vi "标样核查.vi"() -> ()   [LabVIEW 2016, in "斯坦道多参数.lvlib"]
panel:
  out "运行状态":u16(ring) items=["空闲", "水样测试", "标样核查"]
  out "seconds since 1Jan1904":timestamp
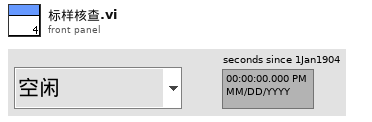
[diagram p1: front panel]
types:
  T1 = cluster{"ph":bool, "DO":bool, "Cond":bool, "Turb":bool, "叶绿素a":bool, "藻密度":bool, "ORP":bool}
  T2 = cluster{"水样数据时间":timestamp, "水样实测值":sgl, "单位":string, "水样数据标识":string, "信号值":sgl, "标样参考值":sgl, "因子编码":string, "探头温度":sgl}
  T3 = cluster{"数据保存间隔":dbl, "保存组数":dbl, "水温标样值":dbl, "pH标样值":dbl, "溶解氧标样值":dbl, "电导率标样值":dbl, "浊度标样值":dbl, "pH启用":bool, "溶解氧启用":bool, "电导率启用":bool, "浊度启用":bool}
  T4 = typedef "LVDateTimeRec.ctl" = cluster{"秒数的小数部分":dbl, "秒":i32, "分":i32, "时":i32, "日":i32, "月":i32, "年":i32, "天数（周）":i32, "天数（年）":i32, "DST":i32}
  T5 = cluster{"温度测量值":sgl, "测量值":sgl, "温度偏移修正值":sgl, "信号值":sgl}
  T6 = cluster{"温度测量值":sgl, "DO%":sgl, "DOmg/L":sgl, "温度偏移修正值":sgl}
  T7 = cluster{"CH":u16, "监测值":dbl, "温度偏移修正值":sgl, "信号值":sgl}
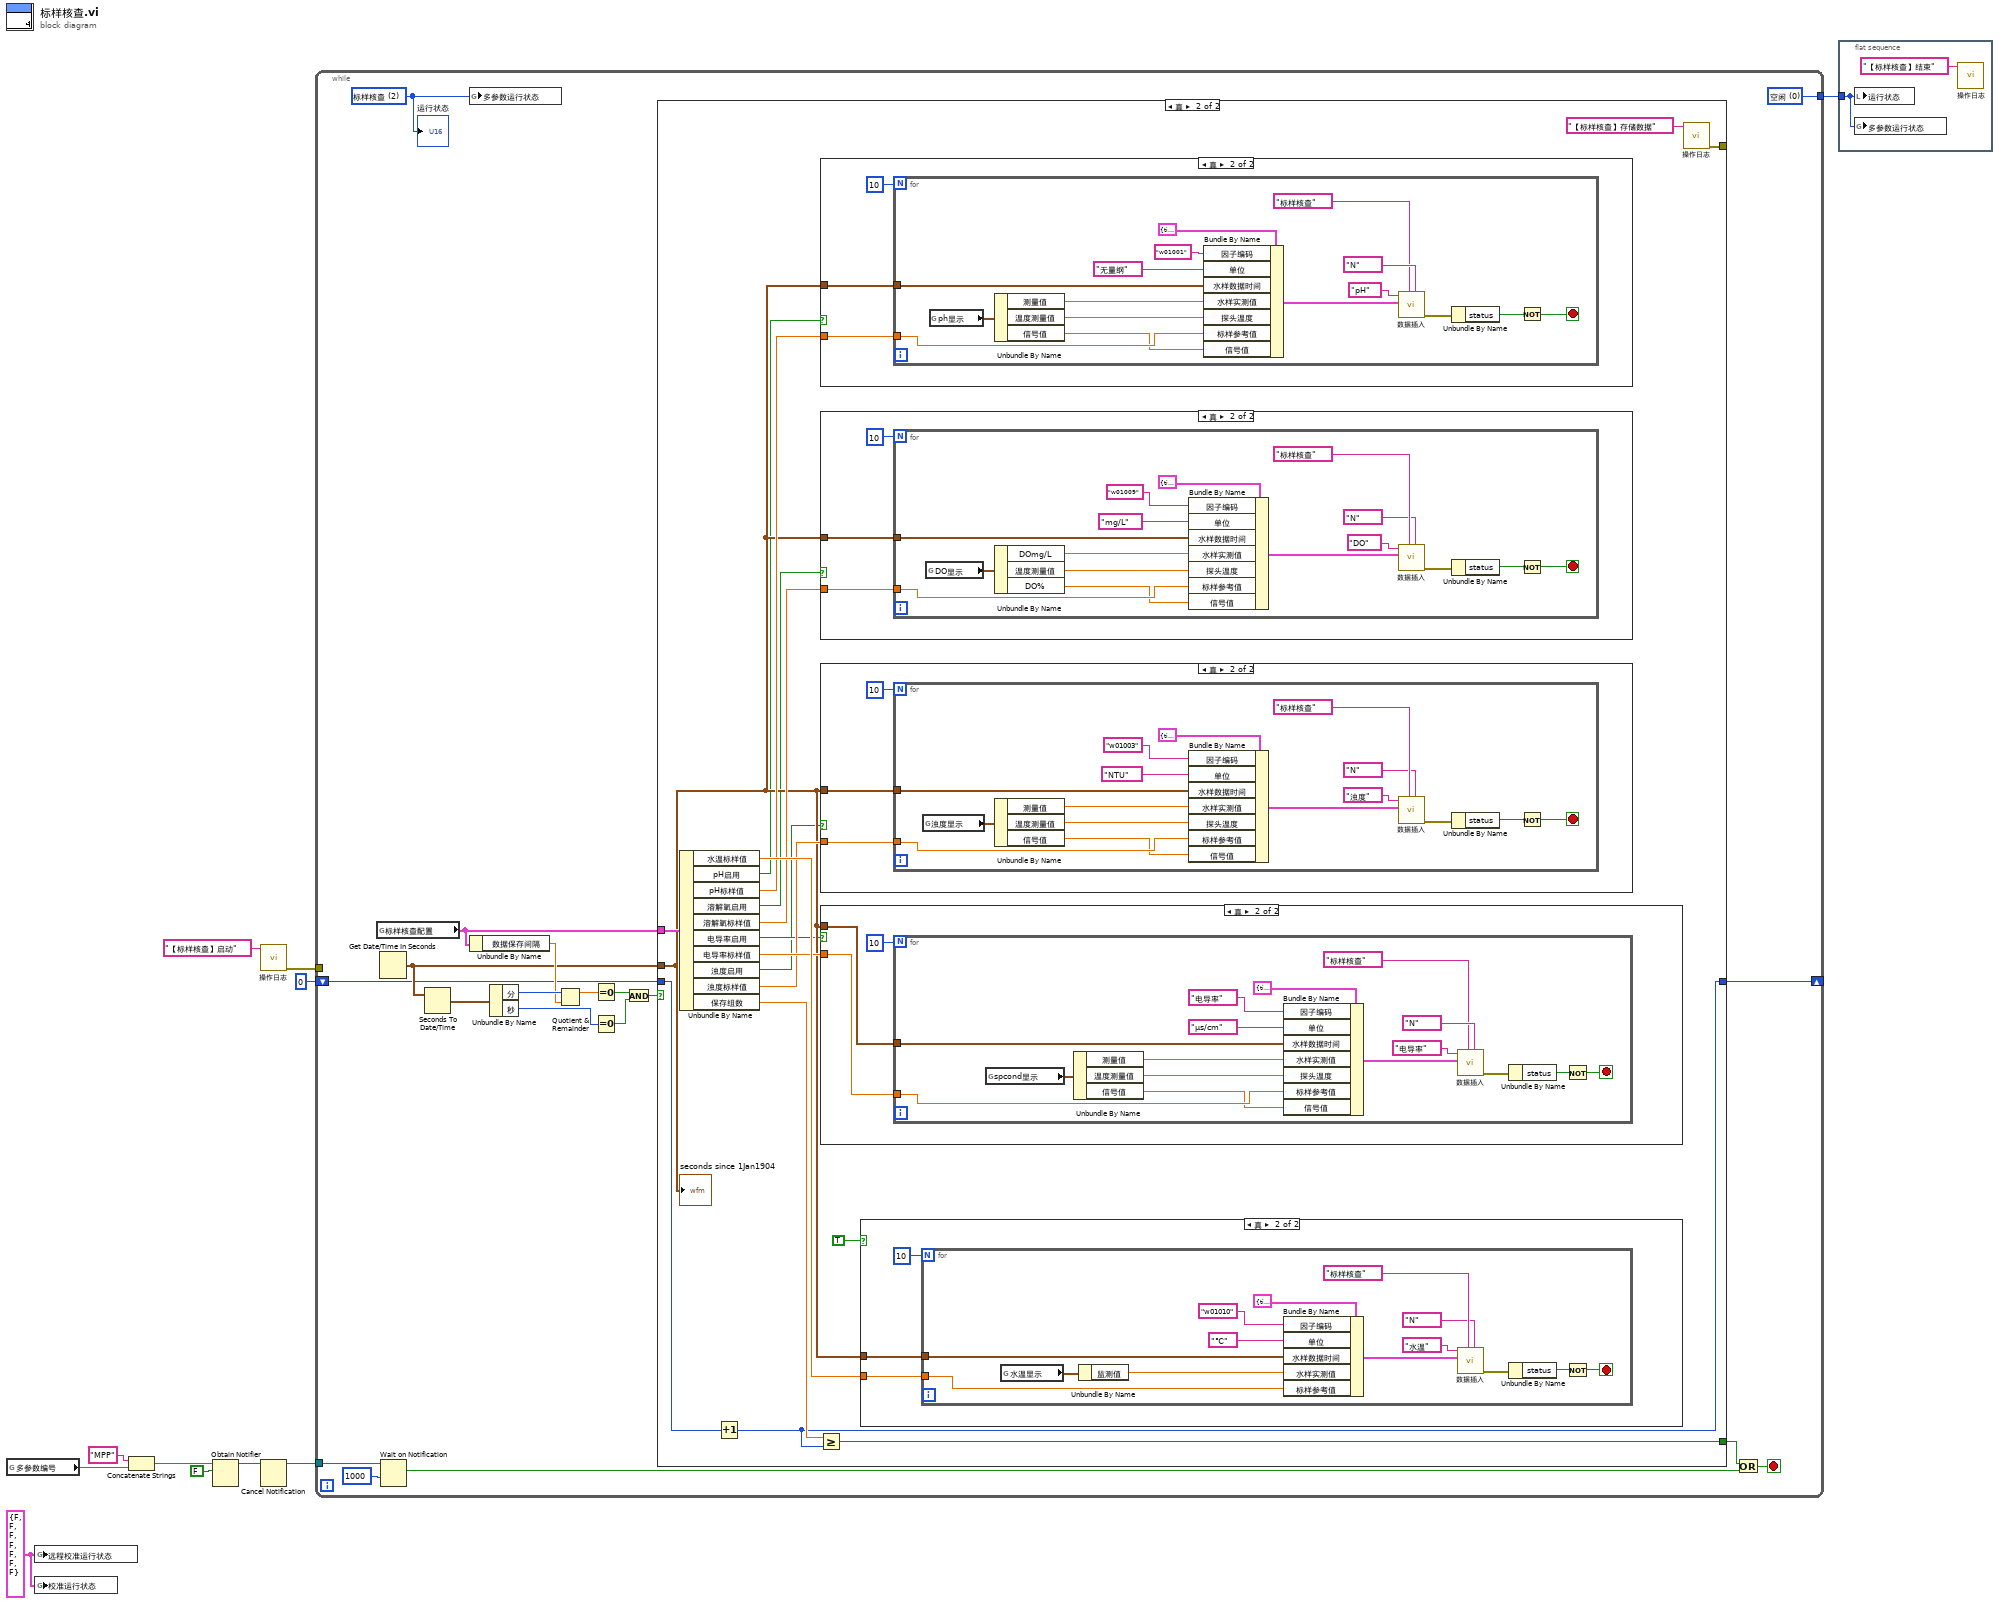
[diagram p0: block diagram]
diagram:
  w2 = T1 {"ph"=FALSE, "DO"=FALSE, "Cond"=FALSE, "Turb"=FALSE, "叶绿素a"=FALSE, "藻密度"=FALSE, "ORP"=FALSE} ("校准运行状态")
  n1 = global read "多参数全局变量.vi" "多参数编号"() -> (w5:string)
  n2 = global write "多参数全局变量.vi" "远程校准运行状态"(w2) -> ()
  n3 = global write "多参数全局变量.vi" "校准运行状态"(w2) -> ()
  n4 = Concatenate Strings("MPP" ("名称（未命名）"), w5) -> (w6:string)
  n5 = Obtain Notifier(name (unnamed)=w6, notification data type=FALSE) -> (notifier out=w9:refnum<notifier>)  [unwired: 2 in, 2 out]
  n6 = call "操作日志.vi"("日志信息"="【标样核查】启动") -> ("error out"=w3:errorcluster)  [unwired: 10 in]
  n7 = Cancel Notification(0:w9) -> (8:w8:refnum<notifier>)  [unwired: 1 in, 2 out]
  n8 = while {
    tunnel: [w21] -> w7
    tunnel: w8 -> [w20]
    tunnel: w3 -> [_]
    shift-right: [w14] -> _
    shift-left: 0 -> [w15]
    stop <- w13 stop-if-true
    w21 = u16 0 items=["空闲", "水样测试", "标样核查"] ("多参数运行状态")
    w17 = u16 2 items=["空闲", "水样测试", "标样核查"] ("多参数运行状态")
    n9 = global read "断电保存变量.vi" "标样核查配置"() -> (w16:T3)
    n10 = Get Date/Time In Seconds() -> (seconds since 1Jan1904=w22:timestamp)
    n11 = Wait on Notification(notifier=w20, timeout in ms (-1)=1000 ("超时毫秒(-1)")) -> (notification=w18:bool)  [unwired: 2 in, 3 out]
    n12 = Seconds To Date/Time(time stamp (now)=w22) -> (date time rec=w30:T4)  [unwired: 1 in]
    n13 = global write "多参数全局变量.vi" "多参数运行状态"(w17) -> ()
    n14 = Unbundle By Name(w16) -> ("数据保存间隔"=w25:dbl)
    n15 = Unbundle By Name(w30) -> ("分"=w26:i32, "秒"=w29:i32)
    n16 = Quotient & Remainder(x=w26, y=w25) -> (x-y*floor(x/y)=w24:dbl)  [unwired: 1 out]
    n17 = Equal To 0?(x=w24) -> (x = 0?=w23:bool)
    n18 = Equal To 0?(x=w29) -> (x = 0?=w28:bool)
    n19 = And(x=w23, y=w28) -> (x .and. y?=w27:bool)
    n20 = case shown="真" w27 {
      tunnel: w16 -> [_ w49]
      tunnel: w22 -> [_ w41]
      tunnel: [_ w42] -> _
      tunnel: w15 -> [w31 w35]
      tunnel: [w31 w33] -> w14
      tunnel: [_ w32] -> w12
      frame False {
      }
      frame True {
        n21 = Unbundle By Name(w49) -> ("水温标样值"=w48:dbl, "pH启用"=w40:bool, "pH标样值"=w47:dbl, "溶解氧启用"=w38:bool, "溶解氧标样值"=w46:dbl, "电导率启用"=w37:bool, "电导率标样值"=w45:dbl, "浊度启用"=w36:bool, "浊度标样值"=w44:dbl, "保存组数"=w34:dbl)
        n22 = Increment(x=w35) -> (x+1=w33:i32)
        n23 = Greater Or Equal?(x=w34, y=w33) -> (x >= y?=w32:bool)
        n24 = case shown="真" w40 {
          tunnel: w47 -> [_ w109]
          tunnel: w41 -> [_ w107]
          frame False {
          }
          frame True {
            n25 = for {
              N: 10 -> [_]
              tunnel: w109 -> [w120]
              tunnel: w107 -> [w113]
              stop <- w114 stop-if-true
              n26 = global read "多参数全局变量.vi" "ph显示"() -> (w119:T5)
              n27 = Unbundle By Name(w119) -> ("测量值"=w118:sgl, "温度测量值"=w117:sgl, "信号值"=w110:sgl)
              n28 = Bundle By Name(cluster=T2 {"水样数据时间"=timestamp(0 s since 1904-01-01), "水样实测值"=0.0, "单位"="", "水样数据标识"="N", "信号值"=0.0, "标样参考值"=0.0, "因子编码"="", "探头温度"=0.0} ("data in"), "因子编码"="w01001", "单位"="无量纲", "水样数据时间"=w113, "水样实测值"=w118, "探头温度"=w117, "标样参考值"=w120, "信号值"=w110) -> (w111:T2)
              n29 = call "数据插入.vi"("数据类型"="N" ("数据标记表"), "测量模式"="标样核查", "data in"=w111, "table输入"="pH") -> ("error out"=w116:errorcluster)  [unwired: 7 in]
              n30 = Unbundle By Name(w116) -> ("status"=w115:bool)
              n31 = Not(x=w115) -> (.not. x?=w114:bool)
            }
          }
        }
        n32 = case shown="真" w38 {
          tunnel: w46 -> [_ w90]
          tunnel: w41 -> [_ w88]
          frame False {
          }
          frame True {
            n33 = for {
              N: 10 -> [_]
              tunnel: w90 -> [w98]
              tunnel: w88 -> [w93]
              stop <- w94 stop-if-true
              n34 = global read "多参数全局变量.vi" "DO显示"() -> (w97:T6)
              n35 = Unbundle By Name(w97) -> ("DOmg/L"=w104:sgl, "温度测量值"=w106:sgl, "DO%"=w91:sgl)
              n36 = Bundle By Name(cluster=T2 {"水样数据时间"=timestamp(0 s since 1904-01-01), "水样实测值"=0.0, "单位"="", "水样数据标识"="N", "信号值"=0.0, "标样参考值"=0.0, "因子编码"="", "探头温度"=0.0} ("data in"), "因子编码"="w01009", "单位"="mg/L", "水样数据时间"=w93, "水样实测值"=w104, "探头温度"=w106, "标样参考值"=w98, "信号值"=w91) -> (w103:T2)
              n37 = call "数据插入.vi"("数据类型"="N" ("数据标记表"), "测量模式"="标样核查", "data in"=w103, "table输入"="DO") -> ("error out"=w96:errorcluster)  [unwired: 7 in]
              n38 = Unbundle By Name(w96) -> ("status"=w95:bool)
              n39 = Not(x=w95) -> (.not. x?=w94:bool)
            }
          }
        }
        n40 = case shown="真" w36 {
          tunnel: w44 -> [_ w52]
          tunnel: w41 -> [_ w50]
          frame False {
          }
          frame True {
            n41 = for {
              N: 10 -> [_]
              tunnel: w52 -> [w62]
              tunnel: w50 -> [w55]
              stop <- w56 stop-if-true
              n42 = global read "多参数全局变量.vi" "浊度显示"() -> (w61:T5)
              n43 = Unbundle By Name(w61) -> ("测量值"=w60:sgl, "温度测量值"=w59:sgl, "信号值"=w53:sgl)
              n44 = Bundle By Name(cluster=T2 {"水样数据时间"=timestamp(0 s since 1904-01-01), "水样实测值"=0.0, "单位"="", "水样数据标识"="N", "信号值"=0.0, "标样参考值"=0.0, "因子编码"="", "探头温度"=0.0} ("data in"), "因子编码"="w01003", "单位"="NTU", "水样数据时间"=w55, "水样实测值"=w60, "探头温度"=w59, "标样参考值"=w62, "信号值"=w53) -> (w67:T2)
              n45 = call "数据插入.vi"("数据类型"="N" ("数据标记表"), "测量模式"="标样核查", "data in"=w67, "table输入"="浊度") -> ("error out"=w58:errorcluster)  [unwired: 7 in]
              n46 = Unbundle By Name(w58) -> ("status"=w57:bool)
              n47 = Not(x=w57) -> (.not. x?=w56:bool)
            }
          }
        }
        n48 = case shown="真" w37 {
          tunnel: w45 -> [_ w71]
          tunnel: w41 -> [_ w69]
          frame False {
          }
          frame True {
            n49 = for {
              N: 10 -> [_]
              tunnel: w71 -> [w82]
              tunnel: w69 -> [w75]
              stop <- w76 stop-if-true
              n50 = global read "多参数全局变量.vi" "spcond显示"() -> (w81:T5)
              n51 = Unbundle By Name(w81) -> ("测量值"=w80:sgl, "温度测量值"=w79:sgl, "信号值"=w72:sgl)
              n52 = Bundle By Name(cluster=T2 {"水样数据时间"=timestamp(0 s since 1904-01-01), "水样实测值"=0.0, "单位"="", "水样数据标识"="N", "信号值"=0.0, "标样参考值"=0.0, "因子编码"="", "探头温度"=0.0} ("data in"), "因子编码"="电导率", "单位"="μs/cm", "水样数据时间"=w75, "水样实测值"=w80, "探头温度"=w79, "标样参考值"=w82, "信号值"=w72) -> (w85:T2)
              n53 = call "数据插入.vi"("数据类型"="N" ("数据标记表"), "测量模式"="标样核查", "data in"=w85, "table输入"="电导率") -> ("error out"=w78:errorcluster)  [unwired: 7 in]
              n54 = Unbundle By Name(w78) -> ("status"=w77:bool)
              n55 = Not(x=w77) -> (.not. x?=w76:bool)
            }
          }
        }
        n56 = case shown="真" TRUE {
          tunnel: w48 -> [_ w128]
          tunnel: w41 -> [_ w127]
          frame False {
          }
          frame True {
            n57 = for {
              N: 10 -> [_]
              tunnel: w128 -> [w136]
              tunnel: w127 -> [w133]
              stop <- w130 stop-if-true
              n58 = global read "多参数全局变量.vi" "水温显示"() -> (w135:T7)
              n59 = Unbundle By Name(w135) -> ("监测值"=w134:dbl)
              n60 = Bundle By Name(cluster=T2 {"水样数据时间"=timestamp(0 s since 1904-01-01), "水样实测值"=0.0, "单位"="", "水样数据标识"="N", "信号值"=0.0, "标样参考值"=0.0, "因子编码"="", "探头温度"=0.0} ("data in"), "因子编码"="w01010", "单位"="℃", "水样数据时间"=w133, "水样实测值"=w134, "标样参考值"=w136) -> (w141:T2)
              n61 = call "数据插入.vi"("数据类型"="N" ("数据标记表"), "测量模式"="标样核查", "data in"=w141, "table输入"="水温") -> ("error out"=w132:errorcluster)  [unwired: 7 in]
              n62 = Unbundle By Name(w132) -> ("status"=w131:bool)
              n63 = Not(x=w131) -> (.not. x?=w130:bool)
            }
          }
        }
        n64 = call "操作日志.vi"("日志信息"="【标样核查】存储数据") -> ("error out"=w42:errorcluster)  [unwired: 10 in]
        "seconds since 1Jan1904" <- w41
      }
    }
    n65 = Or(x=w12, y=w18) -> (x .or. y?=w13:bool)
    "运行状态" <- w17
  }
  n66 = flat-sequence {
    tunnel: w7 -> [w144]
    frame #0 {
      n67 = local write "运行状态"(w144) -> ()
      n68 = global write "多参数全局变量.vi" "多参数运行状态"(w144) -> ()
      n69 = call "操作日志.vi"("日志信息"="【标样核查】结束") -> ()  [unwired: 10 in, 1 out]
    }
  }
